vi "Station Get By ixStation.vi"(8 "error in (no error)":errorcluster, 10 "ixStation (0)":i32, 11 "Connection Refnum":T2) -> (0 "error out":errorcluster, 1 "Instruments on Station":T1[](array[typedef]), 2 "Station Record":T3, 3 "Connection Refnum":T2, 4 "Data Present?":bool)   [LabVIEW 2011]
uses:
  Station Record.ctl
  Instruments/Instrument Record.ctl
  SI.LIB/ODBC/SQL Controls/Connection Refnum.ctl
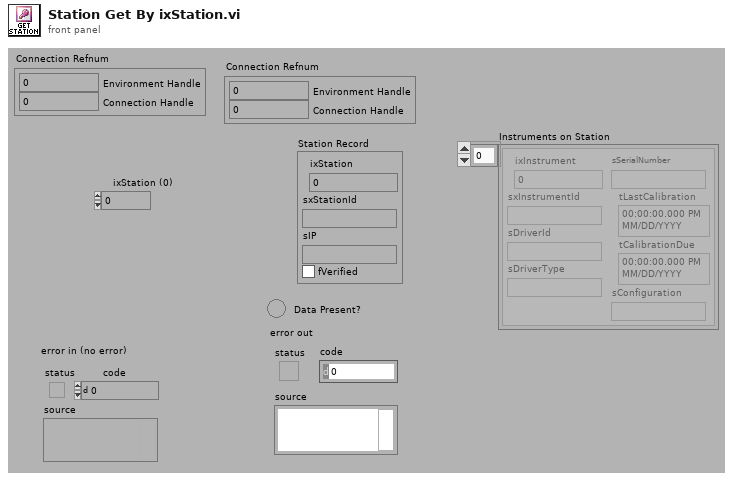
[diagram p1: front panel]
types:
  T1 = typedef "Instrument Record.ctl" = cluster{"ixInstrument":i32, "sxInstrumentId":string, "sDriverId":string, "sDriverType":string, "sSerialNumber":string, "tLastCalibration":timestamp, "tCalibrationDue":timestamp, "sConfiguration":string}
  T2 = typedef "Connection Refnum.ctl" = cluster{"Environment Handle":i32, "Connection Handle":i32}
  T3 = typedef "Station Record.ctl" = cluster{"ixStation":i32, "sxStationId":string, "sIP":string, "fVerified":bool}
  T4 = typedef "Statement Refnum.ctl" = cluster{"Statement Handle":i32, "Parameter Number":u16}
  T5 = typedef "Association Record.ctl" = cluster{"ixAssociation":i32, "iStation":i32, "iInstrument":i32}
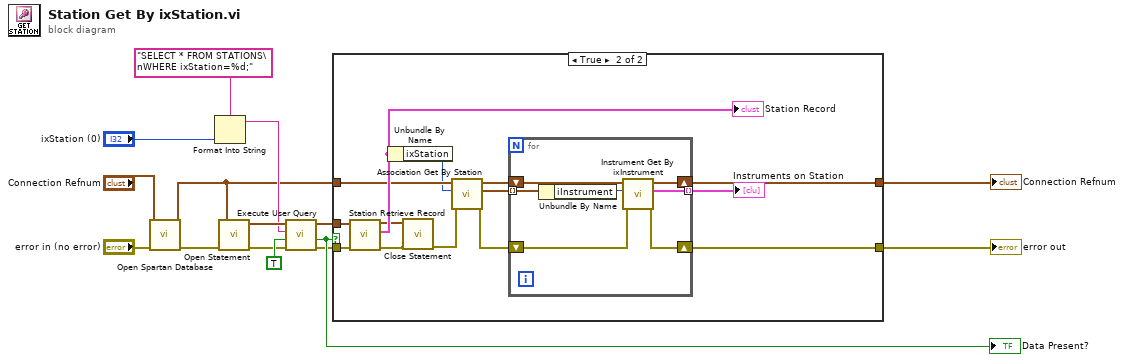
[diagram p0: block diagram]
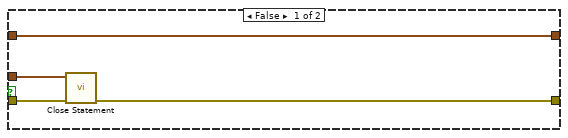
[diagram p2: hidden frame]
diagram:
  n1 = call "Open Spartan Database.vi"("error in (no error)"="error in (no error)", "DB Path (empty - use default)"="Connection Refnum") -> ("error out"=w11:errorcluster, "Connection Refnum"=w3:T2)  [unwired: 8 out]
  n2 = Format Into String(format string="SELECT * FROM STATIONS\nWHERE ixStation=%d;" ("User Query"), "ixStation (0)") -> (resulting string=w6:string)  [unwired: 2 in, 1 out]
  n3 = call "Open Statement.vi"("error in (no error)"=w11, "Connection Refnum"=w3) -> ("error out"=w9:errorcluster, "Statement Refnum"=w8:T4)  [unwired: 4 out]
  n4 = call "Execute User Query.vi"("error in (no error)"=w9, "Return Data? (f)"=TRUE, "User Query"=w6, "Statement Refnum"=w8) -> ("error out"=w14:errorcluster, "Data Present?"=w15:bool, "Statement Refnum"=w13:T4)  [unwired: 1 out]
  "Data Present?" <- w15
  n5 = case shown="True" w15 {
    tunnel: w14 -> [w16 w33]
    tunnel: w13 -> [w17 w32]
    tunnel: [w18 w24] -> w1
    tunnel: w3 -> [w19 w28]
    tunnel: [w19 w26] -> w2
    frame False {
      n6 = call "Close Statement.vi"("error in (no error)"=w16, "Statement Refnum"=w17) -> ("error out"=w18:errorcluster)  [unwired: 5 out]
    }
    frame True {
      n7 = call "Station Retrieve Record.vi"("error in (no error)"=w33, "Statement Refnum"=w32) -> ("error out"=w22:errorcluster, "Station Record"=w31:T3, "Statement Refnum"=w21:T4)  [unwired: 7 out]
      "Station Record" <- w31
      n8 = Unbundle By Name(w31) -> ("ixStation"=w23:i32)
      n9 = call "Close Statement.vi"("error in (no error)"=w22, "Statement Refnum"=w21) -> ("error out"=w20:errorcluster)  [unwired: 5 out]
      n10 = call "Association Get By Station.vi"("error in (no error)"=w20, "iStation (0)"=w23, "Connection Refnum"=w28) -> ("error out"=w25:errorcluster, "Associations"=w30:T5[], "Connection Refnum"=w27:T2)  [unwired: 6 out]
      n11 = for {
        tunnel: w30 -> [w40] mode=indexing
        tunnel: [w39] -> w29 mode=indexing
        shift-right: [w36] -> w26
        shift-left: w27 -> [w37]
        shift-right: [w34] -> w24
        shift-left: w25 -> [w35]
        n12 = Unbundle By Name(w40) -> ("iInstrument"=w38:i32)
        n13 = call "Instrument Get By ixInstrument.vi"("error in (no error)"=w35, "ixInstrument"=w38, "Connection Refnum"=w37) -> ("error out"=w34:errorcluster, "Instrument Record"=w39:T1, "Connection Refnum"=w36:T2)  [unwired: 6 out]
      }
      "Instruments on Station" <- w29
    }
  }
  "error out" <- w1
  "Connection Refnum" <- w2
